vi "create workbook filename (SubVI).vi"(11 "SampleID":string) -> (3 "Excel report workbook file name":path)   [LabVIEW 2015]
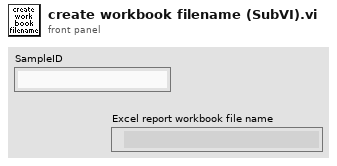
[diagram p1: front panel]
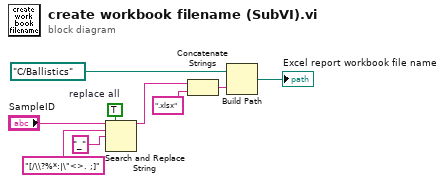
[diagram p0: block diagram]
diagram:
  w2 = TRUE  # replace all
  n1 = Search and Replace String(replace all?=w2, input string="SampleID", search string="[/\\?%*:|\"<>. ;]", replace string="_" ("replace string (\"\")")) -> (result string=w1:string)  [unwired: 4 in, 3 out]
  n2 = Concatenate Strings(w1, ".xlsx" ("string")) -> (w6:string)
  n3 = Build Path(base path=path "C:/Ballistics" ("Custom Template"), name or relative path=w6) -> (appended path=→"Excel report workbook file name":path)
